vi "Start.vi"(8 "error in (no error)":errorcluster, 11 "VISA resource name":refnum<visa-resource-name>) -> (0 "error out":errorcluster, 3 "VISA resource name out":refnum<visa-resource-name>)   [LabVIEW 2012, in "Stanford Research 830.lvlib"]
doc: "Starts or continues a scan. \n\n<B>Note:</B>\n\nThis VI initiates measurements to be placed into the internal buffer. Use this VI only when acquiring multiple points of data."
uses:
  <instrlib>/Stanford Research 830/Stanford Research 830.lvlib
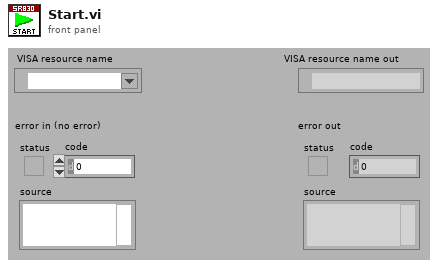
[diagram p1: front panel]
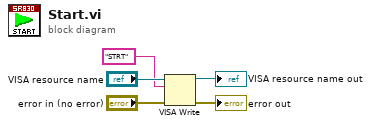
[diagram p0: block diagram]
diagram:
  n1 = VISA Write(VISA resource name="VISA resource name", write buffer="STRT", error in (no error)="error in (no error)") -> (VISA resource name out=→"VISA resource name out":refnum<visa-resource-name>, error out=→"error out":errorcluster)  [unwired: 1 out]
